vi "Piston Pump Test.vi"() -> ()   [LabVIEW 2024]
uses:
  <vilib>/FPGAPlugInAG/cRIO-9068/niLvFpga_Open_cRIO-9068.vi
  <vilib>/rvi/interface/common/dynamic/niFpgaDynamicAddResources.vi
  <vilib>/Utility/error.llb/Error Cluster From Error Code.vi
  <vilib>/rvi/errors/niLvFpgaAdjustHostInterfaceError.vi
  <vilib>/FPGAPlugInAG/Dynamic/niLvFpga_Close_Dynamic.vi
  <vilib>/rvi/interface/nirviOpenFPGA/nirviOpenFPGA.xnode
  FPGA Bitfiles/crio-9068-scan-t_FPGATarget_FPGAMAin_XA2NADVDmlU.lvbitx
  FPGA_MAin.vi
  <vilib>/rvi/interface/nirviReadWriteControl/nirviReadWriteControl.xnode
  <vilib>/rvi/interface/nirviCloseFPGA/nirviCloseFPGA.xnode
  NiFpgaLv.dll
  <vilib>/rvi/interface/Simulation/niFpgaSimulationCallBeginRW.vi
panel:
  in  "Pump Cycle uSec":u32
  in  "Pump Direction":bool
  in  "Pump Enable":bool
  out "error out 2":errorcluster
  in  "stop":bool
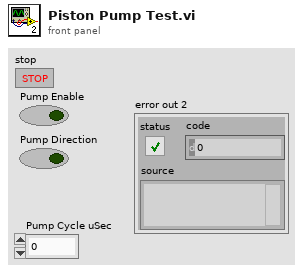
[diagram p1: front panel]
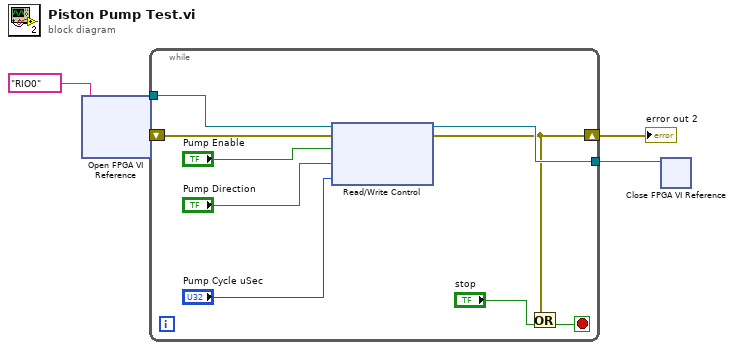
[diagram p0: block diagram]
diagram:
  n1 = xnode "Open FPGA VI Reference"("resource name"=tag "RIO0") -> ("FPGA VI Reference Out"=w4:refnum<k20>, "error out"=w2:errorcluster)  [unwired: 1 in]
  n2 = while {
    tunnel: w4 -> [w14]
    tunnel: [w12] -> w3
    shift-right: [w6] -> w1
    shift-left: w2 -> [w8]
    stop <- w7 stop-if-true
    n3 = xnode "Read/Write Control"("FPGA VI Reference In"=w14, "error in"=w8, "Pump Enable"="Pump Enable", "Pump Direction"="Pump Direction", "Pump Cycle"="Pump Cycle uSec") -> ("FPGA VI Reference Out"=w12:refnum<k20>, "error out"=w6:errorcluster)
    n4 = Or(x=w6, y="stop") -> (x .or. y?=w7:bool)
  }
  "error out 2" <- w1
  n5 = xnode "Close FPGA VI Reference"("FPGA VI Reference In"=w3) -> ()  [unwired: 1 in, 1 out]
